vi "Write CLIP XML Path.vi"(8 "error in (no error)":errorcluster, 10 "CLIP XML Path":path, 11 "RIO Target Configuration in":refnum<class "RIO Target Configuration.lvclass">) -> (0 "error out":errorcluster, 3 "RIO Target Configuration out":refnum<class "RIO Target Configuration.lvclass">)   [LabVIEW 2014, in "RIO Target Configuration.lvclass"]
uses:
  RIO Target Configuration.lvclass
  <vilib>/NI/Configuration Framework/serializable configuration/NISE_CEF_serializable configuration.lvclass
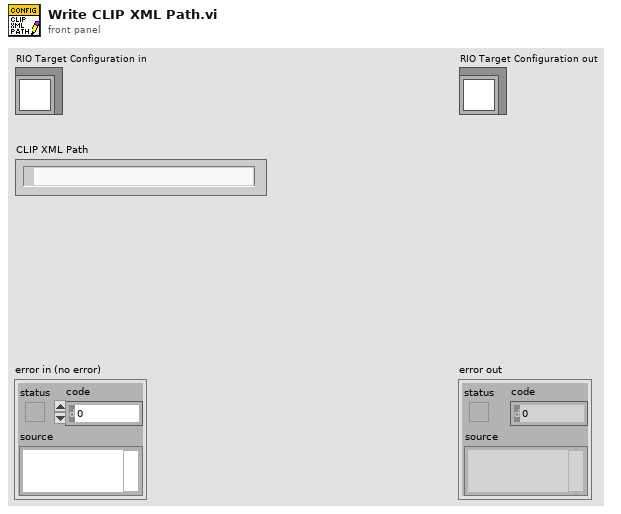
[diagram p1: front panel]
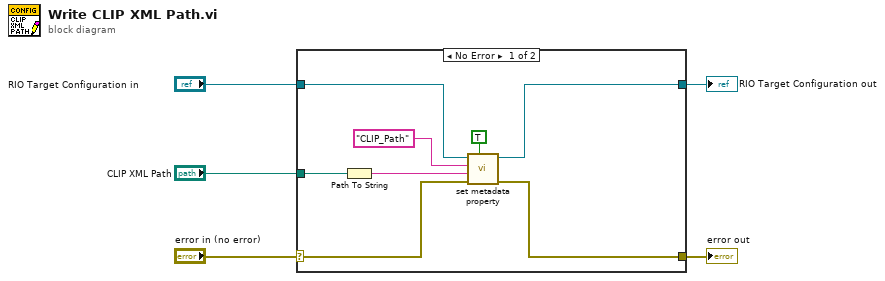
[diagram p0: block diagram]
diagram:
  n1 = case shown="No Error" "error in (no error)" {
    selector: "error in (no error)" -> [w12 w14]
    tunnel: [w8 w14] -> w4
    tunnel: [w6 w15] -> w2
    tunnel: "RIO Target Configuration in" -> [w9 w15]
    tunnel: "CLIP XML Path" -> [w13 _]
    frame No Error {
      n2 = Path To String(path=w13) -> (string=w11:string)
      n3 = call <vilib>:"set metadata property.vi"("overwrite?"=TRUE, "error in"=w12, "value"=w11, "key"="CLIP_Path", "configuration in"=w9) -> ("error out"=w8:errorcluster, "configuration out"=w6:refnum<class "RIO Target Configuration.lvclass">)  [unwired: 5 in]
    }
    frame Error {
    }
  }
  "error out" <- w4
  "RIO Target Configuration out" <- w2
